vi "Wait For Logging Command.vi"(8 "error in (no error)":errorcluster, 9 "timeout in ms (0)":i32 format="%d ms", 11 "Logging Interface in":refnum<class "Logging Interface.lvclass">) -> (0 "error out":errorcluster, 2 "command":T1={"Command"=enum."Log Plugin State", "Parameters"={"arg1"=0, "arg2"=0}}, 3 "Logging Interface out":refnum<class "Logging Interface.lvclass">, 4 "# elements":u32)   [LabVIEW 2017, in "DSF Core.lvlib" / "Logging Interface.lvclass"]
uses:
  Logging Interface.lvclass
  C:/Git/DSF/Core/Classes/Interface/Interface.lvclass
  Command Data.ctl
  Command.ctl
  Parameters.ctl
  Dispatcher/Command Timeout.vi
  Interface.lvclass
  DSF Core.lvlib
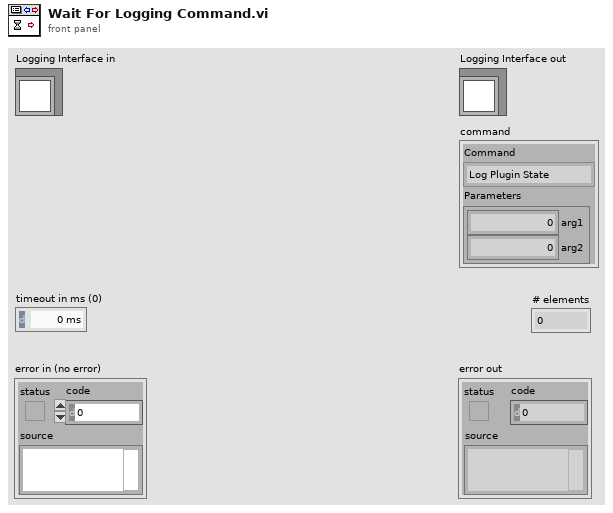
[diagram p1: front panel]
types:
  T1 = typedef "DSF Core.lvlib/Logging Interface.lvclass/Command Data.ctl" = cluster{"Command":T2, "Parameters":T3}
  T2 = typedef "DSF Core.lvlib/Logging Interface.lvclass/Command.ctl" = enum8{"Idle", "Start", "Log Framework State", "Log Plugin State", "Log Dispatcher State", "Shutdown"}
  T3 = typedef "DSF Core.lvlib/Logging Interface.lvclass/Parameters.ctl" = cluster{"arg1":u64, "arg2":u64}
  T4 = typedef "DSF Core.lvlib/Interface.lvclass/RT FIFO Data.ctl" = cluster{"Command":u8, "Parameters":T5}
  T5 = typedef "DSF Core.lvlib/Interface.lvclass/RT FIFO Parameters.ctl" = cluster{"arg1":u64, "arg2":u64}
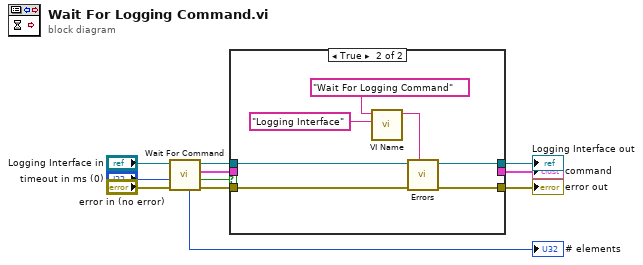
[diagram p0: block diagram]
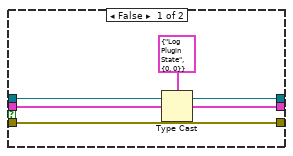
[diagram p2: hidden frame]
diagram:
  n1 = call "Wait For Command.vi"("error in (no error)"="error in (no error)", "timeout in ms (0)"="timeout in ms (0)", "Interface in"="Logging Interface in") -> ("error out"=w2:errorcluster, "timed out?"=w5:bool, "command"=w6:T4, "Interface out"=w4:refnum<class "Logging Interface.lvclass">, "# elements"=→"# elements":u32)  [unwired: 4 in]
  n2 = case shown="True" w5 {
    tunnel: [w14 _] -> w11
    tunnel: w6 -> [w13 _]
    tunnel: w4 -> [w16 w23]
    tunnel: [w16 w21] -> w3
    tunnel: w2 -> [w12 w22]
    tunnel: [w12 w20] -> w1
    frame False {
      n3 = Type Cast(type=T1 {"Command"=enum."Log Plugin State", "Parameters"={"arg1"=0, "arg2"=0}} ("Logging Command"), x=w13) -> (*(type *) &x=w14:T1)
    }
    frame True {
      n4 = call "VI Name.vi"("class name (\"\")"="Logging Interface" ("class name (\"\")"), "vi name"="Wait For Logging Command" ("error source vi name")) -> ("full VI name"=w18:string)  [unwired: 9 in]
      n5 = call-poly "Errors.vi"("error source vi name"=w18, "error in (no error)"=w22, "Interface in"=w23) -> ("error out"=w20:errorcluster, "Interface out"=w21:refnum<class "Logging Interface.lvclass">)  [unwired: 7 in]
    }
  }
  "error out" <- w1
  "Logging Interface out" <- w3
  "command" <- w11
